vi "CS_schleife.vi"   [LabVIEW 2019]
uses:
  Global/Global Variables/global.vi
  Instrument_Setup.vi
  Monitors/Utility/Monitor Communication/sub-vis/16T_Open_Queue.vi
  Global/Global Variables/Data_Display_global.vi
  Monitors/Utility/Monitor Communication/sub-vis/16T_Split_Cluster.vi
  Monitors/Utility/Monitor Communication/sub-vis/16T_Queue_Commands.vi
  Monitors/Utility/Monitor Communication/sub-vis/20T_Open_Queue.vi
  Monitors/Utility/Monitor Communication/sub-vis/20T_Split_Cluster.vi
  Monitors/Utility/Monitor Communication/sub-vis/20T_Queue_Commands.vi
types:
  T1 = typedef "16T-Cluster.ctl" = cluster{"Clamp":bool, "Switch Heater":bool, "Go to Zero":bool, "Go to set":bool, "Go to Hold":bool, "Clamped":bool, "Quenched":bool, "Rate limit":bool, "Persistent":bool, "Hold":bool, "Set":bool, "Zero":bool, "Magnet (T)":dbl, "Leads (T)":dbl, "Magnet T (K)":dbl, "Switch":bool, "Setpoint (T)":dbl, "Rate (T/min)":dbl, "Select":bool, "Sweeping":bool}
  T2 = typedef "16T_Control.ctl" = cluster{"Clamp":bool, "Switch Heater":bool, "Go to Zero":bool, "Go to Set":bool, "Go to Hold":bool, "Setpoint (T)":dbl, "Rate (T/min)":dbl, "Set Rate":bool}
  T3 = typedef "15T-Cluster.ctl" = cluster{"Magnet (T)":dbl, "Leads (T)":dbl, "Setpoint (T)":dbl, "Rate (T/min)":dbl, "Set":bool, "Zero":bool, "Hold":bool, "Go to zero":bool, "Go to Hold":bool, "Go to Set":bool, "Clamp":bool, "Switch Heater":bool, "Rate limit":bool, "Switch":bool, "Clamped":bool, "Persistent":bool, "Quenched":bool, "Sweeping":bool, "Select":bool}
  T4 = typedef "15T-Control.ctl" = cluster{"Setpoint (T)":dbl, "Rate (T/min)":dbl, "Go to zero":bool, "Go to Hold":bool, "Go to Set":bool, "Clamp":bool, "Switch Heater":bool}
  T5 = typedef "20T_Cluster.ctl" = cluster{"Clamp":bool, "Switch Heater":bool, "Go to Zero":bool, "Go to set":bool, "Go to Hold":bool, "Clamped":bool, "Quenched":bool, "Rate limit":bool, "Persistent":bool, "Hold":bool, "Set":bool, "Zero":bool, "Magnet (T)":dbl, "Leads (T)":dbl, "Magnet T (K)":dbl, "Switch":bool, "Target (T)":dbl, "Setpoint (T)":dbl, "Rate (T/min)":dbl, "Switch Heater 2":bool, "Set Rate":bool}
  T6 = typedef "20T_Control.ctl" = cluster{"Clamp":bool, "Switch Heater":bool, "Go to Zero":bool, "Go to Set":bool, "Go to Hold":bool, "Setpoint (T)":dbl, "Rate (T/min)":dbl, "Set Rate":bool}
  T7 = typedef "5T-Cluster.ctl" = cluster{"Go to set":bool, "Go to Zero":bool, "Clamp":bool, "Go to Hold":bool, "Clamped ":bool, "Quenched 2":bool, "Rate limit 2":bool, "Magnet (T)":dbl, "Leads (T)":dbl, "Rate (T/min)":dbl, "Sweeping":bool, "Setpoint":dbl, "Set":bool, "Zero":bool, "Hold":bool, "Clamp":bool}
  T8 = typedef "5T_Control.ctl" = cluster{"Rate (T/min)":dbl, "Setpoint":dbl, "Go to set":bool, "Go to Zero":bool, "Clamp":bool, "Go to Hold":bool, "Set Rate":bool}
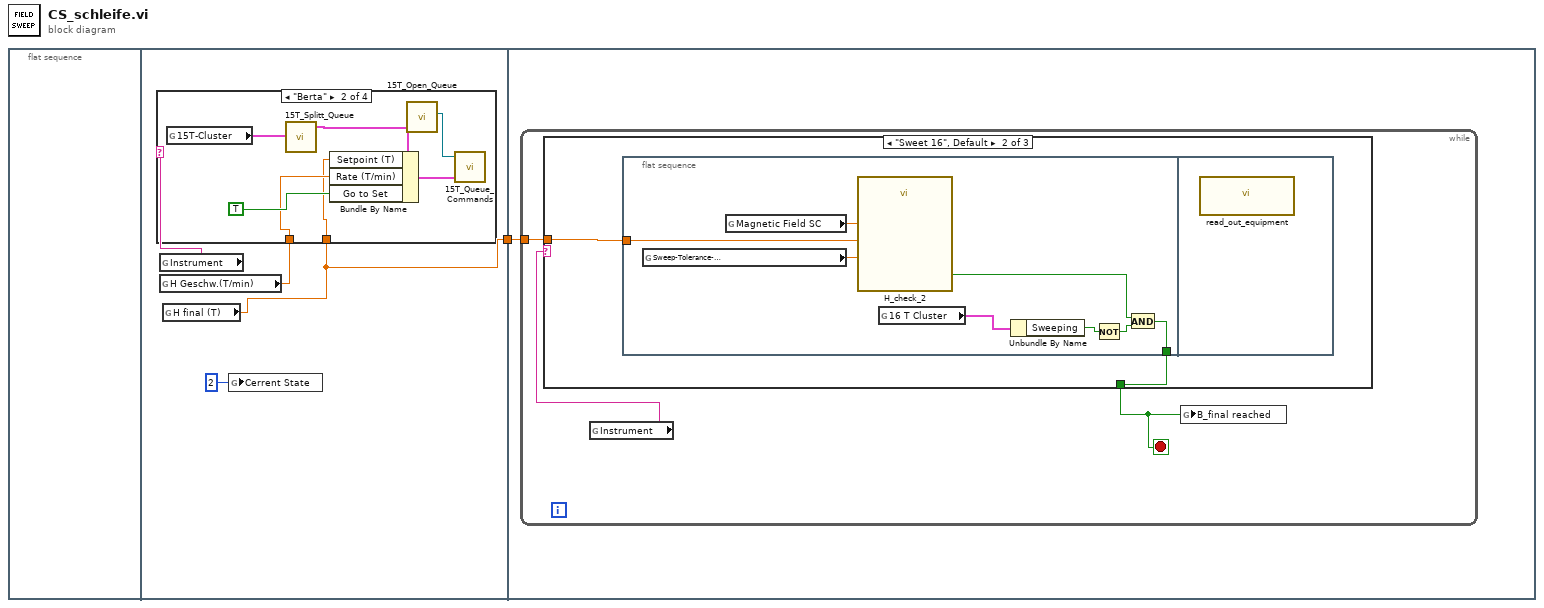
[diagram p0: block diagram]
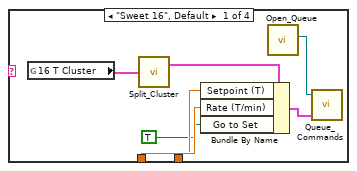
[diagram p2: hidden frame]
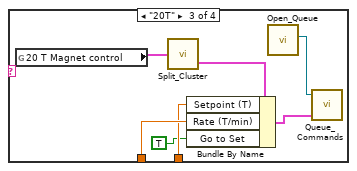
[diagram p3: hidden frame]
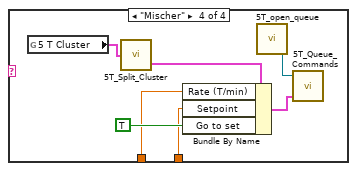
[diagram p4: hidden frame]
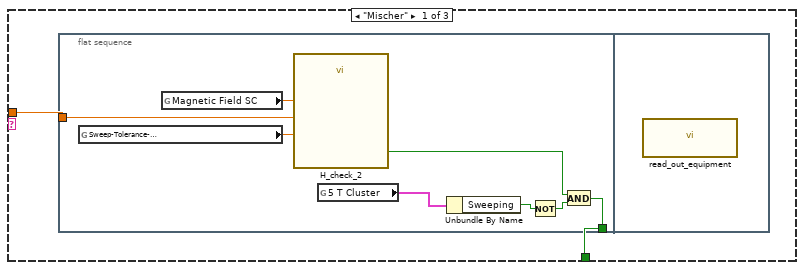
[diagram p5: hidden frame]
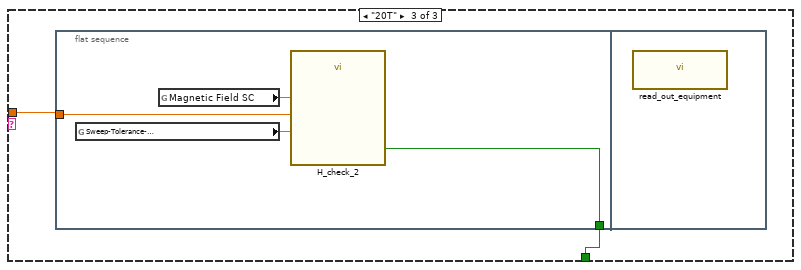
[diagram p6: hidden frame]
diagram:
  n1 = flat-sequence {
    tunnel: [w3] -> w1
    tunnel: w1 -> [w34]
    frame #0 {
    }
    frame #1 {
      n2 = global read "Instrument_Setup.vi" "Instrument"() -> (w2:string)
      n3 = global read "global.vi" "H Geschw.(T/min)"() -> (w4:dbl)
      n4 = global read "global.vi" "H final (T)"() -> (w3:dbl)
      n5 = case shown="\"Berta\"" w2 {
        tunnel: w4 -> [w10 w14 w22 w28]
        tunnel: w3 -> [w9 w13 w21 w27]
        frame "Sweet 16", Default {
          n6 = global read "Data_Display_global.vi" "16 T Cluster"() -> (w11:T1)
          n7 = call-poly "Split_Cluster.vi"("16 T Magnet control"=w11) -> ("16 T Magnet control"=w8:T2)  [unwired: 1 out]
          n8 = Bundle By Name(cluster=w8, "Setpoint (T)"=w9, "Rate (T/min)"=w10, "Go to Set"=TRUE) -> (w7:T2)
          n9 = call-poly "Open_Queue.vi"() -> ("queue out"=w12:refnum<queue>)  [unwired: 10 in, 1 out]
          n10 = call-poly "Queue_Commands.vi"("16 T Magnet control"=w7, "16T Queue"=w12) -> ()  [unwired: 1 in, 1 out]
        }
        frame "Berta" {
          n11 = global read "Data_Display_global.vi" "15T-Cluster"() -> (w18:T3)
          n12 = call "15T_Splitt_Queue.vi"("15T-Cluster"=w18) -> ("15T-Control"=w17:T4)  [unwired: 1 in, 1 out]
          n13 = Bundle By Name(cluster=w17, "Setpoint (T)"=w13, "Rate (T/min)"=w14, "Go to Set"=TRUE) -> (w15:T4)
          n14 = call "15T_Open_Queue.vi"() -> ("queue out"=w19:refnum<queue>)  [unwired: 10 in, 1 out]
          n15 = call "15T_Queue_Commands.vi"("15T-Control"=w15, "15T Queue"=w19) -> ()  [unwired: 1 in, 1 out]
        }
        frame "20T" {
          n16 = global read "Data_Display_global.vi" "20 T Magnet control"() -> (w25:T5)
          n17 = call-poly "Split_Cluster.vi"("20 T Cluster"=w25) -> ("20 T Control"=w23:T6)  [unwired: 1 out]
          n18 = Bundle By Name(cluster=w23, "Setpoint (T)"=w21, "Rate (T/min)"=w22, "Go to Set"=TRUE) -> (w24:T6)
          n19 = call-poly "Open_Queue.vi"() -> ("queue out"=w26:refnum<queue>)  [unwired: 10 in, 1 out]
          n20 = call-poly "Queue_Commands.vi"("20 T Control"=w24, "20T Queue"=w26) -> ()  [unwired: 1 in, 1 out]
        }
        frame "Mischer" {
          n21 = global read "Data_Display_global.vi" "5 T Cluster"() -> (w33:T7)
          n22 = call "5T_Split_Cluster.vi"("5 T Cluster"=w33) -> ("5T Control"=w32:T8)  [unwired: 1 out]
          n23 = Bundle By Name(cluster=w32, "Rate (T/min)"=w28, "Setpoint"=w27, "Go to set"=TRUE) -> (w31:T8)
          n24 = call "5T_open_queue.vi"() -> ("queue out"=w30:refnum<queue>)  [unwired: 10 in, 1 out]
          n25 = call "5T_Queue_Commands.vi"("5T Control"=w31, "5T Queue"=w30) -> ()  [unwired: 1 in, 1 out]
        }
      }
      n26 = global write "global.vi" "Cerrent State"(2) -> ()
    }
    frame #2 {
      n27 = while {
        tunnel: w34 -> [w36]
        stop <- w37 stop-if-true
        n28 = global read "Instrument_Setup.vi" "Instrument"() -> (w35:string)
        n29 = case shown="\"Sweet 16\", Default" w35 {
          tunnel: [w38 w49 w58] -> w37
          tunnel: w36 -> [w39 w48 w59]
          frame "Mischer" {
            n30 = flat-sequence {
              tunnel: [w42] -> w38
              tunnel: w39 -> [w45]
              frame #0 {
                n31 = global read "Instrument_Setup.vi" "Sweep-Tolerance-\nMagnetic-Field"() -> (w47:dbl)
                n32 = global read "Data_Display_global.vi" "Magnetic Field SC"() -> (w46:dbl)
                n33 = call "H_check_2.vi"("Sweep\nTolerance %"=w47, "H_in"=w46, "H_target (K)"=w45) -> ("= H target"=w43:bool)  [unwired: 8 in]
                n34 = global read "Data_Display_global.vi" "5 T Cluster"() -> (w44:T7)
                n35 = Unbundle By Name(w44) -> ("Sweeping"=w40:bool)
                n36 = Not(x=w40) -> (.not. x?=w41:bool)
                n37 = And(x=w43, y=w41) -> (x .and. y?=w42:bool)
              }
              frame #1 {
                n38 = call "read_out_equipment.vi"() -> ()  [unwired: 1 in]
              }
            }
          }
          frame "Sweet 16", Default {
            n39 = flat-sequence {
              tunnel: [w52] -> w49
              tunnel: w48 -> [w55]
              frame #0 {
                n40 = global read "Instrument_Setup.vi" "Sweep-Tolerance-\nMagnetic-Field"() -> (w57:dbl)
                n41 = global read "Data_Display_global.vi" "Magnetic Field SC"() -> (w56:dbl)
                n42 = call "H_check_2.vi"("Sweep\nTolerance %"=w57, "H_in"=w56, "H_target (K)"=w55) -> ("= H target"=w53:bool)  [unwired: 8 in]
                n43 = global read "Data_Display_global.vi" "16 T Cluster"() -> (w54:T1)
                n44 = Unbundle By Name(w54) -> ("Sweeping"=w50:bool)
                n45 = Not(x=w50) -> (.not. x?=w51:bool)
                n46 = And(x=w53, y=w51) -> (x .and. y?=w52:bool)
              }
              frame #1 {
                n47 = call "read_out_equipment.vi"() -> ()  [unwired: 1 in]
              }
            }
          }
          frame "20T" {
            n48 = flat-sequence {
              tunnel: [w60] -> w58
              tunnel: w59 -> [w61]
              frame #0 {
                n49 = global read "Instrument_Setup.vi" "Sweep-Tolerance-\nMagnetic-Field"() -> (w63:dbl)
                n50 = global read "Data_Display_global.vi" "Magnetic Field SC"() -> (w62:dbl)
                n51 = call "H_check_2.vi"("Sweep\nTolerance %"=w63, "H_in"=w62, "H_target (K)"=w61) -> ("= H target"=w60:bool)  [unwired: 8 in]
              }
              frame #1 {
                n52 = call "read_out_equipment.vi"() -> ()  [unwired: 1 in]
              }
            }
          }
        }
        n53 = global write "Data_Display_global.vi" "B_final reached"(w37) -> ()
      }
    }
  }
